vi "myRIO v1.0 Write PWM.vi"(8 "error in (no error)":errorcluster, 9 "PWM Configuration In":T1, 10 "Channel":T2, 11 "myRIO Ref In":T3) -> (0 "error out":errorcluster, 2 "PWM Configuration Out":T1, 3 "myRIO Ref Out":T3)   [LabVIEW 2021]
uses:
  <vilib>/myRIO/Common/Instrument Driver Framework/Utilities/typedefs/myRIO v1.0 Reference.ctl
  <vilib>/myRIO/Common/Instrument Driver Framework/Utilities/typedefs/Generic FPGA Reference.ctl
  <vilib>/myRIO/Common/Instrument Driver Framework/myRIO v1.0/PWM/typedefs/PWM Channels Enum.ctl
  <vilib>/myRIO/Common/Instrument Driver Framework/myRIO v1.0/PWM/typedefs/PWM Configuration v1.0.ctl
  <vilib>/myRIO/Common/Instrument Driver Framework/myRIO v1.0/PWM/typedefs/PWM Channels FPGA Reference.ctl
  <vilib>/myRIO/Common/Instrument Driver Framework/Utilities/vis/Calculate Clock Settings.vi
  <vilib>/myRIO/Common/Instrument Driver Framework/Utilities/vis/Calculate TOP (Phase Correct Mode).vi
  <vilib>/myRIO/Common/Instrument Driver Framework/Utilities/vis/Calculate TOP (Normal Mode).vi
  <vilib>/myRIO/Common/Instrument Driver Framework/Utilities/vis/Calculate Frequency (Phase Correct Mode).vi
  <vilib>/myRIO/Common/Instrument Driver Framework/Utilities/vis/Calculate Frequency (Normal Mode).vi
  <vilib>/rvi/errors/niLvFpgaAdjustHostInterfaceError.vi
  <vilib>/rvi/interface/nirviReadWriteControl/nirviReadWriteControl.xnode
  <vilib>/rvi/interface/Simulation/niFpgaSimulationCallBeginRW.vi
  NiFpgaLv.dll
panel:
  # "This VI writes a value to each output compare register (OCCRA and OCCRB) for a particular PWM channel. The output compare values are used to define the duty cycles of the PWM outputs. Please see Block Diagram for details."
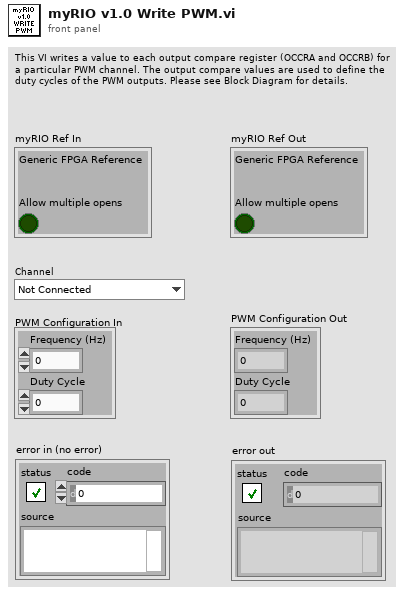
[diagram p1: front panel]
types:
  T1 = typedef "PWM Configuration v1.0.ctl" = cluster{"Frequency (Hz)":dbl, "Duty Cycle":dbl}
  T2 = typedef "PWM Channels Enum.ctl" = enum16{"Not Connected", "C/PWM0", "C/PWM1", "A/PWM0", "A/PWM1", "A/PWM2", "A/PWM3", "A/PWM4", "A/PWM5", "A/PWM6", "A/PWM7", "A/PWM8", "A/PWM9", "A/PWM10", "A/PWM11", "A/PWM12", "A/PWM13", "A/PWM14", "A/PWM15", "A/PWM16", "A/PWM17", "A/PWM18", "A/PWM19", "B/PWM0", "B/PWM1", "B/PWM2", "B/PWM3", "B/PWM4", "B/PWM5", "B/PWM6", "B/PWM7", "B/PWM8", "B/PWM9", "B/PWM10", "B/PWM11", "B/PWM12", "B/PWM13", "B/PWM14", "B/PWM15", "B/PWM16", "B/PWM17", "B/PWM18", "B/PWM19", "PWM/PWM0", "PWM/PWM1", "PWM/PWM2", "PWM/PWM3", "PWM/PWM4", "PWM/PWM5", "PWM/PWM6", "PWM/PWM7", "PWM/PWM8", "PWM/PWM9"}
  T3 = typedef "myRIO v1.0 Reference.ctl" = cluster{"Generic FPGA Reference":T4, "Allow multiple opens":bool}
  T4 = typedef "Generic FPGA Reference.ctl" = refnum<k20>
  T5 = typedef "PWM Channels FPGA Reference.ctl" = refnum<k20>
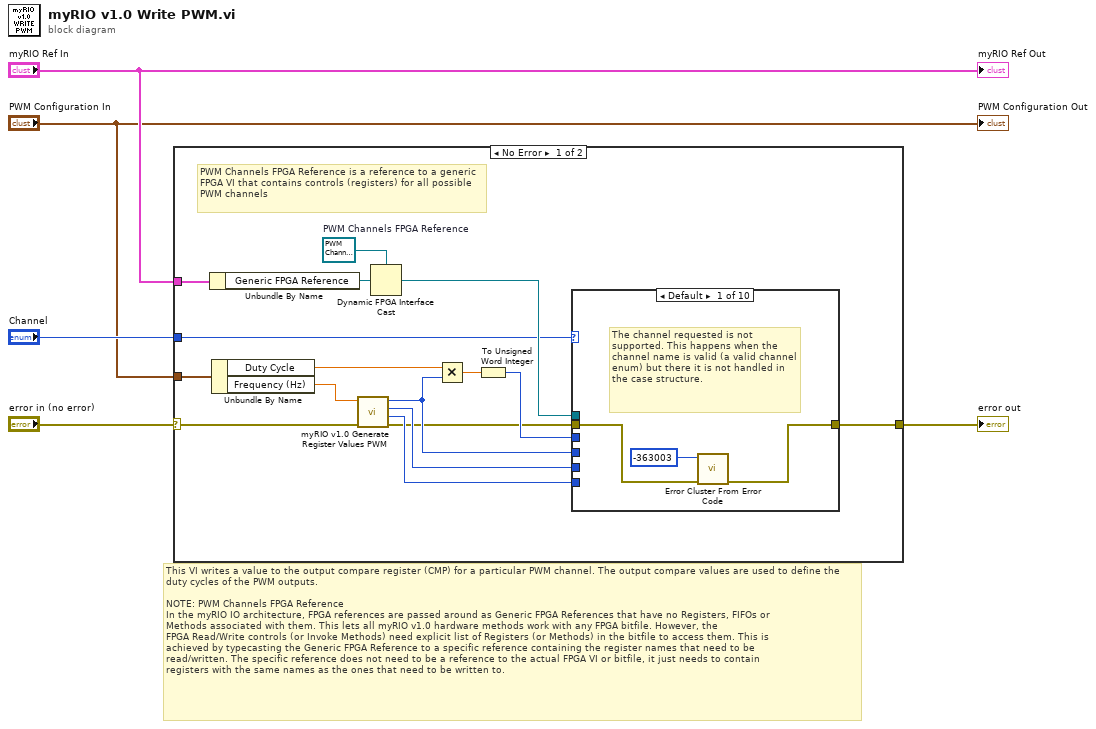
[diagram p0: block diagram]
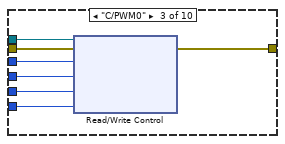
[diagram p3: hidden frame]
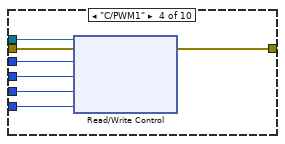
[diagram p4: hidden frame]
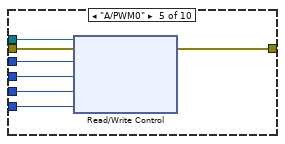
[diagram p5: hidden frame]
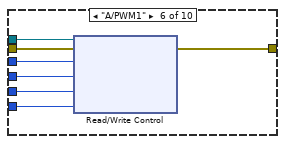
[diagram p6: hidden frame]
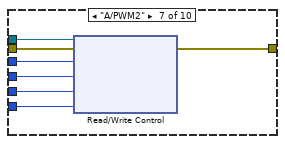
[diagram p7: hidden frame]
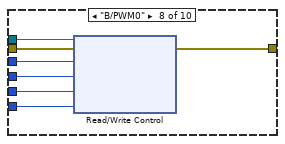
[diagram p8: hidden frame]
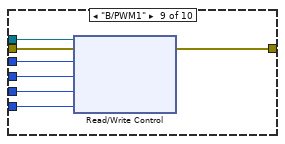
[diagram p9: hidden frame]
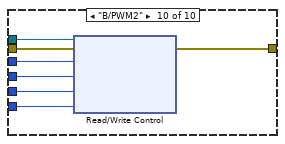
[diagram p10: hidden frame]
diagram:
  # "This VI writes a value to the output compare register (CMP) for a particular PWM channel. The output compare values are used to define the duty cycles of the PWM outputs.\n\nNOTE: PWM Channels FPGA Reference\nIn the myRIO IO architecture, FPGA references are passed around as Generic FPGA References that have no Registers, FIFOs or\nMethods associated with them. This lets all myRIO v1.0 hardware methods work with any FPGA bitfile. However, the \nFPGA Read/Write controls (or Invoke Methods) need explicit list of Registers (or Methods) in the bitfile to access them. This is \nachieved by typecasting the Generic FPGA Reference to a specific reference containing the register names that need to be \nread/written. The specific reference does not need to be a reference to the actual FPGA VI or bitfile, it just needs to contain \nregisters with the same names as the ones that need to be written to."
  n1 = case shown="No Error" "error in (no error)" {
    selector: "error in (no error)" -> [w9 w82]
    tunnel: "myRIO Ref In" -> [w19 _]
    tunnel: [w18 w82] -> w4
    tunnel: "Channel" -> [w17 _]
    tunnel: "PWM Configuration In" -> [w7 _]
    frame No Error {
      w21 = T5 refnum  # PWM Channels FPGA Reference
      # "PWM Channels FPGA Reference is a reference to a generic FPGA VI that contains controls (registers) for all possible PWM channels"
      n2 = Unbundle By Name(w19) -> ("Generic FPGA Reference"=w16:T4)
      n3 = Unbundle By Name(w7) -> ("Duty Cycle"=w15:dbl, "Frequency (Hz)"=w6:dbl)
      n4 = call <vilib>:"myRIO v1.0 Generate Register Values PWM.vi"("error in (no error)"=w9, "Frequency (Hz)"=w6) -> ("error out"=w8:errorcluster, "PWM.CS"=w10:u8, "PWM.CNFG"=w11:u8, "PWM.MAX"=w12:u16)  [unwired: 5 in, 1 out]
      n5 = Dynamic FPGA Interface Cast(Session In=w21, Type=w16) -> (Session Out=w20:T5)
      n6 = Multiply(x=w15, y=w12) -> (x*y=w14:dbl)
      n7 = To Unsigned Word Integer(number=w14) -> (unsigned 16bit integer=w13:u16)
      n8 = case shown="Default" w17 {
        tunnel: w8 -> [w22 w25 w32 w39 w46 w53 w60 w67 w74 w81]
        tunnel: [w23 w25 w31 w38 w45 w52 w59 w66 w73 w80] -> w18
        tunnel: w20 -> [_ _ w30 w37 w44 w51 w58 w65 w72 w79]
        tunnel: w13 -> [_ _ w29 w36 w43 w50 w57 w64 w71 w78]
        tunnel: w12 -> [_ _ w26 w33 w40 w47 w54 w62 w68 w75]
        tunnel: w11 -> [_ _ w28 w34 w41 w48 w55 w61 w69 w76]
        tunnel: w10 -> [_ _ w27 w35 w42 w49 w56 w63 w70 w77]
        frame Default {
          # "The channel requested is not supported. This happens when the channel name is valid (a valid channel enum) but there it is not handled in the case structure."
          n9 = call <vilib>:"Error Cluster From Error Code.vi"("error in (no error)"=w22, "error code (0)"=-363003) -> ("error out"=w23:errorcluster)  [unwired: 7 in]
        }
        frame "Not Connected" {
        }
        frame "C/PWM0" {
          n10 = xnode "Read/Write Control"("FPGA VI Reference In"=w30, "error in"=w32, "PWM.C_0.CMP"=w29, "PWM.C_0.MAX"=w26, "PWM.C_0.CNFG"=w28, "PWM.C_0.CS"=w27) -> ("error out"=w31:errorcluster)  [unwired: 1 out]
        }
        frame "C/PWM1" {
          n11 = xnode "Read/Write Control"("FPGA VI Reference In"=w37, "error in"=w39, "PWM.C_1.CMP"=w36, "PWM.C_1.MAX"=w33, "PWM.C_1.CNFG"=w34, "PWM.C_1.CS"=w35) -> ("error out"=w38:errorcluster)  [unwired: 1 out]
        }
        frame "A/PWM0" {
          n12 = xnode "Read/Write Control"("FPGA VI Reference In"=w44, "error in"=w46, "PWM.A_0.CMP"=w43, "PWM.A_0.MAX"=w40, "PWM.A_0.CNFG"=w41, "PWM.A_0.CS"=w42) -> ("error out"=w45:errorcluster)  [unwired: 1 out]
        }
        frame "A/PWM1" {
          n13 = xnode "Read/Write Control"("FPGA VI Reference In"=w51, "error in"=w53, "PWM.A_1.CMP"=w50, "PWM.A_1.MAX"=w47, "PWM.A_1.CNFG"=w48, "PWM.A_1.CS"=w49) -> ("error out"=w52:errorcluster)  [unwired: 1 out]
        }
        frame "A/PWM2" {
          n14 = xnode "Read/Write Control"("FPGA VI Reference In"=w58, "error in"=w60, "PWM.A_2.CMP"=w57, "PWM.A_2.MAX"=w54, "PWM.A_2.CNFG"=w55, "PWM.A_2.CS"=w56) -> ("error out"=w59:errorcluster)  [unwired: 1 out]
        }
        frame "B/PWM0" {
          n15 = xnode "Read/Write Control"("FPGA VI Reference In"=w65, "error in"=w67, "PWM.B_0.CMP"=w64, "PWM.B_0.MAX"=w62, "PWM.B_0.CNFG"=w61, "PWM.B_0.CS"=w63) -> ("error out"=w66:errorcluster)  [unwired: 1 out]
        }
        frame "B/PWM1" {
          n16 = xnode "Read/Write Control"("FPGA VI Reference In"=w72, "error in"=w74, "PWM.B_1.CMP"=w71, "PWM.B_1.MAX"=w68, "PWM.B_1.CNFG"=w69, "PWM.B_1.CS"=w70) -> ("error out"=w73:errorcluster)  [unwired: 1 out]
        }
        frame "B/PWM2" {
          n17 = xnode "Read/Write Control"("FPGA VI Reference In"=w79, "error in"=w81, "PWM.B_2.CMP"=w78, "PWM.B_2.MAX"=w75, "PWM.B_2.CNFG"=w76, "PWM.B_2.CS"=w77) -> ("error out"=w80:errorcluster)  [unwired: 1 out]
        }
      }
    }
    frame Error {
      # "Nothing to do since there was an incoming error."
    }
  }
  "error out" <- w4
  "myRIO Ref Out" <- "myRIO Ref In"
  "PWM Configuration Out" <- "PWM Configuration In"
